vi "ParseLogHTML.vi"(3 "vi name":string="_LVROS__LVROS_Node_Server_vi") -> (0 "Text":string="Node: /LVROS\n Port: 57299\n__________________________________\nServer Information\nServer: _LVROS__LVROS_Node_Server_vi.vi\nCurrent time: 12:04:13.518 PM\nClient Servers\nServer: Publisher: /junk:57059\nCurrent time: 12:04:03.537 PM\n__________________________________\n\nStarting Server /LVROS__LVROS_Node_Server_vi_Log.html\nNo Error\n\nRegistered Server /junk__LVROS_Publisher_Server_vi_Log.html with master\n\n\n        Method name: Publisher \nTime stamp: 12:04:03.534 PM \nText sent To Robot \nPOST /RPC2 HTTP/1.1\nHost: http://127.0.0.1:11311\nContent-Type: text/xml\nContent-Length: 395\n\n<?xml version='1.0'?>\n<methodCall>\n <methodName>registerPublisher</methodName>\n <params>\n   <param><value><string>/LVROS</string>\n   </value>\n   </param>\n   <param><value><string>/junk</string>\n   </value>\n   </param>\n   <param><value><string>/LVROS/string</string>\n   </value>\n   </param>\n   <param><value><string>http://127.0.0.1:57299</string>\n   </value>\n   </param>\n </params>\n</methodCall>\n\nText replied From Robot \n\nHTTP/1.1 200 OK\nServer: BaseHTTP/Labview\nDate: Thu, 19 Mar 2015 12:04:03 EST\nContent-Type: text/xml\nContent-Length: 402\n\n<?xml version='1.0'?>\n<methodResponse>\n <params>\n  <param>\n   <value>\n    <array>\n     <data>\n      <value><int>1</int>\n      </value>\n      <value><string>Registered [/LVROS] as publisher of [/junk]</string>\n      </value>\n      <value>\n       <array>\n        <data>\n         \n        </data>\n       </array>\n      </value>\n     </data>\n    </array>\n   </value>\n  </param>\n </params>\n</methodResponse>\nUnregistered Server /junk__LVROS_Publisher_Server_vi_Log.html with master\n\n\n        Method name: unregisterPublisher \nTime stamp: 12:04:12.205 PM \nText sent To Robot \nPOST /RPC2 HTTP/1.1\nHost: http://127.0.0.1:11311\nContent-Type: text/xml\nContent-Length: 307\n\n<?xml version='1.0'?>\n<methodCall>\n <methodName>unregisterPublisher</methodName>\n <params>\n   <param><value><string>/LVROS</string> </value> </param>\n   <param><value><string>/junk</string> </value> </param>\n   <param><value><string>http://127.0.0.1:57299</string> </value> </param>\n </params>\n</methodCall>\n\nText replied From Robot \n\nHTTP/1.1 200 OK\nServer: BaseHTTP/Labview\nDate: Thu, 19 Mar 2015 12:04:12 EST\nContent-Type: text/xml\nContent-Length: 270\n\n<?xml version='1.0'?>\n<methodResponse><params><param><value><array><data><value><int>1</int> </value> <value><string>Unregistered[/LVROS] as provider of [/junk]</string> </value> <value><int>1</int> </value> </data> </array> </value> </param> </params> </methodResponse>\nServer /LVROS__LVROS_Node_Server_vi_Log.html Closed\nNo Error\n\n", 1 "2D Picture":picture)   [LabVIEW 2014]
doc: "Parses an HTML log and returns a color coded picture for use in ROSNode.vi as well as parsed text"
panel:
  out "String":string="<!DOCTYPE html>\n<html>\n<head>\n<style type='text/css'>\n.tab {margin-left:40px;}\n</style>\n\n</head>\n<script language=\"JavaScript\" type=\"text/javascript\">\n<!-- Copyright 2005, Sandeep Gangadharan -->\n<!-- For more free scripts go to http://www.sivamdesign.com/scripts/ -->\n<!--\nif (document.getElementById) {\ndocument.writeln('<style type=\"text/css\"><!--')\ndocument.writeln('.texter {display:none} @media print {.texter {display:block;}}')\ndocument.writeln('//--></style>') }\n\nfunction openClose(theID) {\nif (document.getElementById(theID).style.display == \"block\") { document.getElementById(theID).style.display = \"none\" }\nelse { document.getElementById(theID).style.display = \"block\" } }\n// -->\n</script>\n\n<body>\n<a href='index.html'>Return to console</a>\n<!----- start server ----->\n<center><font color = \"black\" size=5>Node: /LVROS</font></center><br>\n<center><font color = \"black\" size=3>Port: 57299</font></center> \n<!----- end server ----->\n \n<div onClick=\"openClose('server')\" \nstyle=\"cursor:hand; cursor:pointer\">\n<font color='blue'>Server Information</font></div>\n<div id=\"server\" class=\"texter\"> \n<p class='tab'>Server: _LVROS__LVROS_Node_Server_vi.vi<br>\nCurrent time: 12:04:13.518 PM<br>\n</p></div>\n<!----- start clients ----->\n<div onClick=\"openClose('clients')\" style=\"cursor:hand; cursor:pointer\">\n<font color='blue'>Client Servers</font></div>\n <div id=\"clients\" class=\"texter\"><p class='tab'>\n\n<a href=\"_junk__LVROS_Publisher_Server_vi_Log.html\">Server: Publisher: /junk:57059</a><br>\nCurrent time: 12:04:03.537 PM<br></p>\n</div>\n<!----- end clients ----->\n<hr>\n<!----- start log ----->      \n<div onClick=\"openClose('log1')\" \nstyle=\"cursor:hand; cursor:pointer\">\n<font color=\"green\">Starting Server /LVROS__LVROS_Node_Server_vi_Log.html</font></div>\n<div id=\"log1\" class=\"texter\">\n<font size=\"2\">\n<p class='tab'></font></p><br>\n<font size =\"2\" color=\"green\" class='tab'>No Error</font><br><br>\n      </div>\n<div onClick=\"openClose('log4')\"\n style=\"cursor:hand; cursor:pointer\">\n<font color=\"green\">Registered Server /junk__LVROS_Publisher_Server_vi_Log.html with master</font></div>\n<div id=\"log4\" class=\"texter\">\n<p class='tab'><font size=\"2\">\n<br>\n        Method name: Publisher <br>\nTime stamp: 12:04:03.534 PM <br><br>\nText sent To Robot </p><br>\n<p class='tab'><font size =\"1\" color=\"purple\"><xmp>POST /RPC2 HTTP/1.1\nHost: http://127.0.0.1:11311\nContent-Type: text/xml\nContent-Length: 395\n\n<?xml version='1.0'?>\n<methodCall>\n <methodName>registerPublisher</methodName>\n <params>\n   <param><value><string>/LVROS</string>\n   </value>\n   </param>\n   <param><value><string>/junk</string>\n   </value>\n   </param>\n   <param><value><string>/LVROS/string</string>\n   </value>\n   </param>\n   <param><value><string>http://127.0.0.1:57299</string>\n   </value>\n   </param>\n </params>\n</methodCall></xmp></font></p><br>\n <br>\n<p class='tab'>Text replied From Robot </p><br>\n<font size =\"1\" color=\"orange\"><xmp>HTTP/1.1 200 OK\nServer: BaseHTTP/Labview\nDate: Thu, 19 Mar 2015 12:04:03 EST\nContent-Type: text/xml\nContent-Length: 402\n\n<?xml version='1.0'?>\n<methodResponse>\n <params>\n  <param>\n   <value>\n    <array>\n     <data>\n      <value><int>1</int>\n      </value>\n      <value><string>Registered [/LVROS] as publisher of [/junk]</string>\n      </value>\n      <value>\n       <array>\n        <data>\n         \n        </data>\n       </array>\n      </value>\n     </data>\n    </array>\n   </value>\n  </param>\n </params>\n</methodResponse></xmp></font><br>\n<font size =\"2\" color=\"green\" class='tab'>No Error</font><br><br>\n<p class='tab'><font color='green'>Notified /junk__LVROS_Publisher_Server_vi_Log.html Server of registration</font></p><br>\n</font>\n      </div>\n<div onClick=\"openClose('log6')\"\n style=\"cursor:hand; cursor:pointer\">\n<font color=\"green\">Unregistered Server /junk__LVROS_Publisher_Server_vi_Log.html with master</font></div>\n<div id=\"log6\" class=\"texter\">\n<p class='tab'><font size=\"2\">\n<br>\n        Method name: unregisterPublisher <br>\nTime stamp: 12:04:12.205 PM <br><br>\nText sent To Robot </p><br>\n<p class='tab'><font size =\"1\" color=\"purple\"><xmp>POST /RPC2 HTTP/1.1\nHost: http://127.0.0.1:11311\nContent-Type: text/xml\nContent-Length: 307\n\n<?xml version='1.0'?>\n<methodCall>\n <methodName>unregisterPublisher</methodName>\n <params>\n   <param><value><string>/LVROS</string> </value> </param>\n   <param><value><string>/junk</string> </value> </param>\n   <param><value><string>http://127.0.0.1:57299</string> </value> </param>\n </params>\n</methodCall></xmp></font></p><br>\n <br>\n<p class='tab'>Text replied From Robot </p><br>\n<font size =\"1\" color=\"orange\"><xmp>HTTP/1.1 200 OK\nServer: BaseHTTP/Labview\nDate: Thu, 19 Mar 2015 12:04:12 EST\nContent-Type: text/xml\nContent-Length: 270\n\n<?xml version='1.0'?>\n<methodResponse><params><param><value><array><data><value><int>1</int> </value> <value><string>Unregistered[/LVROS] as provider of [/junk]</string> </value> <value><int>1</int> </value> </data> </array> </value> </param> </params> </methodResponse></xmp></font><br>\n<font size =\"2\" color=\"green\" class='tab'>No Error</font><br><br>\n<p class='tab'><font color='green'>Notified /junk__LVROS_Publisher_Server_vi_Log.html Server of unregistration</font></p><br>\n</font>\n      </div>\n<div onClick=\"openClose('log8')\" \nstyle=\"cursor:hand; cursor:pointer\">\n<font color=\"green\">Server /LVROS__LVROS_Node_Server_vi_Log.html Closed</font></div>\n<div id=\"log8\" class=\"texter\">\n<font size=\"2\">\n<p class='tab'></font></p><br>\n<font size =\"2\" color=\"green\" class='tab'>No Error</font><br><br>\n      </div>\n<!----- end log ----->\n\n\n</body>\n</html>"
  # "Still does not get all of the lines in the response...."
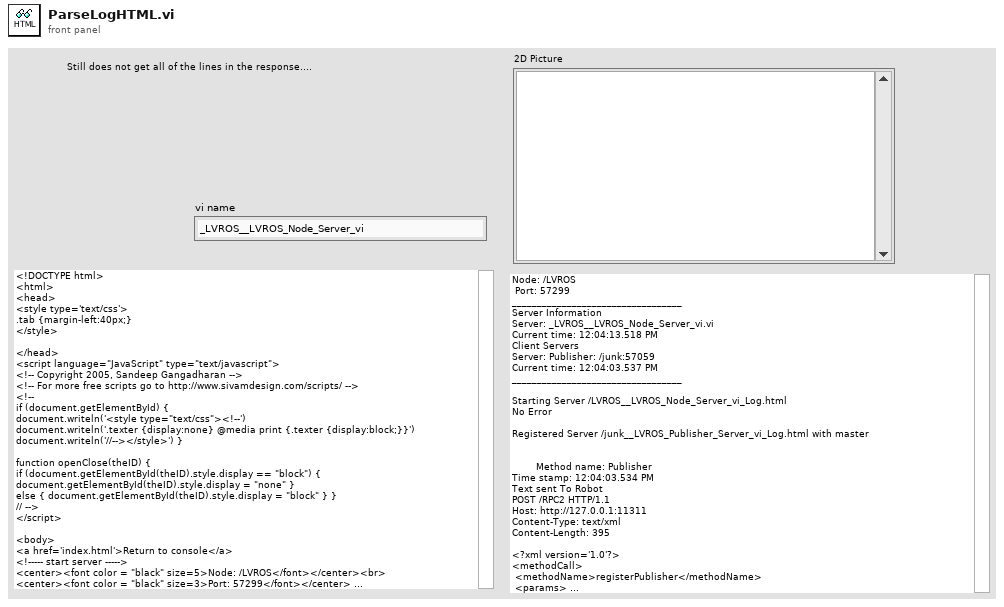
[diagram p1: front panel]
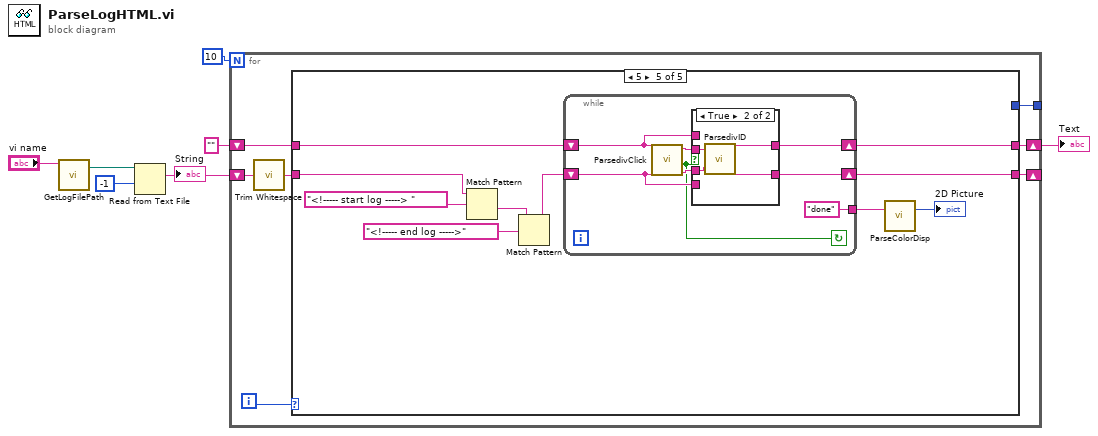
[diagram p0: block diagram]
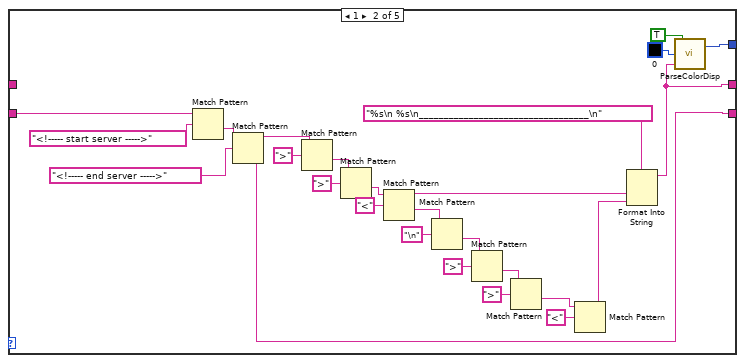
[diagram p3: hidden frame]
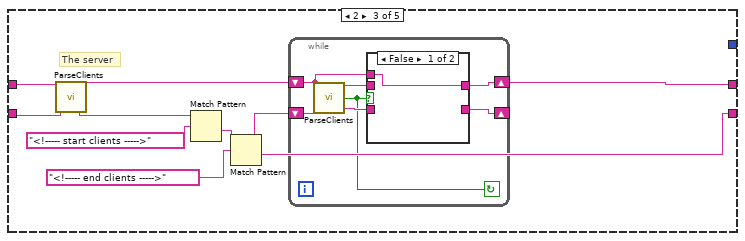
[diagram p4: hidden frame]
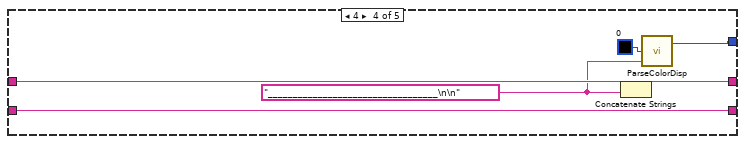
[diagram p6: hidden frame]
diagram:
  n1 = call "GetLogFilePath.vi"("Server name"="vi name") -> ("LogPath"=w6:path)  [unwired: 1 in, 1 out]
  n2 = Read from Text File(file (use dialog)=w6, count=-1) -> (text=w2:string)  [unwired: 2 in, 3 out]
  "String" <- w2
  n3 = for {
    N: 10 -> [_]
    shift-right: [w14] -> w4
    shift-left: "" -> [w11]
    shift-right: [w10] -> _
    shift-left: w2 -> [w12]
    tunnel: [w9] -> _
    i -> [w13]
    n4 = call <vilib>:"Trim Whitespace.vi"("string"=w12) -> ("trimmed string"=w8:string)  [unwired: 1 in]
    n5 = case shown="5" w13 {
      tunnel: w8 -> [w15 w42 w47 w67 w73]
      tunnel: [w16 w18 w43 w66 w71] -> w14
      tunnel: w11 -> [w16 _ w48 w68 w78]
      tunnel: [w15 w22 w49 w67 w77] -> w10
      tunnel: [_ w20 _ w65 _] -> w9
      frame 0, Default {
      }
      frame 1 {
        n6 = Match Pattern(string=w42, regular expression="<!----- start server ----->") -> (after substring=w24:string)  [unwired: 1 in, 3 out]
        n7 = Match Pattern(string=w24, regular expression="<!----- end server ----->") -> (before substring=w21:string, after substring=w22:string)  [unwired: 1 in, 2 out]
        n8 = Match Pattern(string=w21, regular expression=">") -> (after substring=w38:string)  [unwired: 1 in, 3 out]
        n9 = Match Pattern(string=w38, regular expression=">") -> (after substring=w36:string)  [unwired: 1 in, 3 out]
        n10 = Match Pattern(string=w36, regular expression="<") -> (before substring=w26:string, after substring=w34:string)  [unwired: 1 in, 2 out]
        n11 = Match Pattern(string=w34, regular expression="\n") -> (after substring=w28:string)  [unwired: 1 in, 3 out]
        n12 = Match Pattern(string=w28, regular expression=">") -> (after substring=w31:string)  [unwired: 1 in, 3 out]
        n13 = Match Pattern(string=w31, regular expression=">") -> (after substring=w33:string)  [unwired: 1 in, 3 out]
        n14 = Match Pattern(string=w33, regular expression="<") -> (before substring=w25:string)  [unwired: 1 in, 3 out]
        n15 = Format Into String(format string="%s\n %s\n__________________________________\n" ("regular expression"), w26, w25) -> (resulting string=w18:string)  [unwired: 2 in, 1 out]
        n16 = call "ParseColorDisp.vi"("text"=w18, "text color(black)"=u32 0, "Init?"=TRUE) -> ("picture out"=w20:picture)  [unwired: 1 in]
      }
      frame 2 {
        # "The server"
        n17 = call "ParseClients.vi"("Text in"=w48, "HTML in"=w47) -> ("Text out"=w45:string, "HTML out"=w46:string)  [unwired: 1 out]
        n18 = Match Pattern(string=w46, regular expression="<!----- start clients ----->") -> (after substring=w51:string)  [unwired: 1 in, 3 out]
        n19 = Match Pattern(string=w51, regular expression="<!----- end clients ----->") -> (before substring=w44:string, after substring=w49:string)  [unwired: 1 in, 2 out]
        n20 = while {
          shift-right: [w58] -> w43
          shift-left: w45 -> [w53]
          shift-right: [w56] -> _
          shift-left: w44 -> [w59]
          stop <- w54 continue-if-true
          n21 = call "ParseClients.vi"("Text in"=w53, "HTML in"=w59) -> ("Text out"=w57:string, "success?"=w54:bool, "HTML out"=w55:string)
          n22 = case shown="False" w54 {
            tunnel: [w60 w62] -> w58
            tunnel: w57 -> [_ w62]
            tunnel: [_ w61] -> w56
            tunnel: w55 -> [_ w61]
            tunnel: w53 -> [w60 _]
            frame False {
            }
            frame True {
            }
          }
        }
      }
      frame 4 {
        w63 = "__________________________________\n\n" ("regular expression")
        n23 = Concatenate Strings(w68, w63) -> (w66:string)
        n24 = call "ParseColorDisp.vi"("text"=w63, "text color(black)"=u32 0) -> ("picture out"=w65:picture)  [unwired: 2 in]
      }
      frame 5 {
        n25 = Match Pattern(string=w73, regular expression="<!----- start log -----> ") -> (after substring=w74:string)  [unwired: 1 in, 3 out]
        n26 = Match Pattern(string=w74, regular expression="<!----- end log ----->") -> (before substring=w72:string)  [unwired: 1 in, 3 out]
        n27 = while {
          shift-right: [w84] -> w71
          shift-left: w78 -> [w82]
          shift-right: [w83] -> w77
          shift-left: w72 -> [w81]
          tunnel: ["done"] -> w69
          stop <- w80 continue-if-true
          n28 = call "ParsedivClick.vi"("Text in"=w82, "HTML in"=w81) -> ("Text out"=w86:string, "success?"=w80:bool, "HTML out"=w85:string)  [unwired: 1 out]
          n29 = case shown="True" w80 {
            tunnel: w86 -> [_ w92]
            tunnel: w85 -> [_ w91]
            tunnel: [w88 w90] -> w84
            tunnel: [w87 w89] -> w83
            tunnel: w82 -> [w88 _]
            tunnel: w81 -> [w87 _]
            frame False {
            }
            frame True {
              n30 = call "ParsedivID.vi"("Text in"=w92, "HTML in"=w91) -> ("Test out"=w90:string, "HTML out"=w89:string)  [unwired: 1 in]
            }
          }
        }
        n31 = call "ParseColorDisp.vi"("text"=w69) -> ("picture out"=→"2D Picture":picture)  [unwired: 3 in]
      }
    }
  }
  "Text" <- w4
